vi "20.04.2025 class.vi"() -> ()   [LabVIEW 2020]
panel:
  in  "second subarray 3":dbl[][][](array[numeric])
  out "output array":dbl[](array[numeric])
  out "reversed array 2":dbl[](array[numeric])
  out "second subarray":dbl[](array[numeric])
  out "first subarray":dbl[](array[numeric])
  out "reversed array":dbl[](array[numeric])
  in  "Array":dbl[](array[numeric])
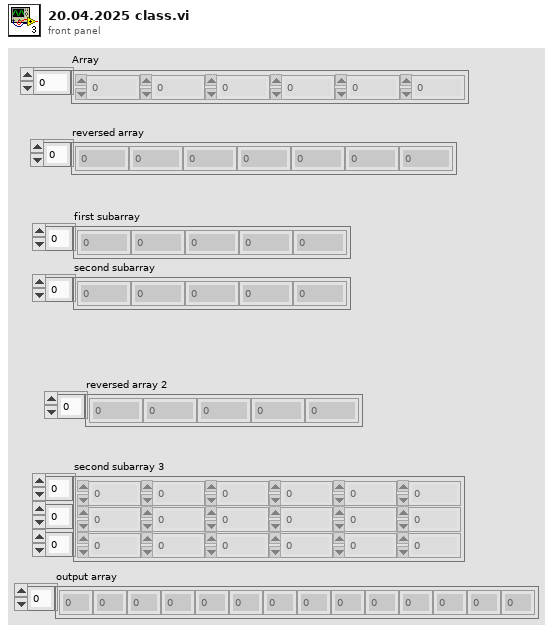
[diagram p1: front panel]
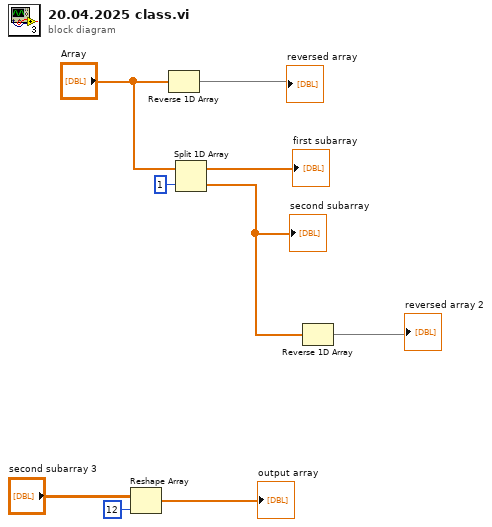
[diagram p0: block diagram]
diagram:
  n1 = Reshape Array "Reshape Array"("second subarray 3", 12 ("dimension size")) -> (→"output array":dbl[])
  n2 = Reverse 1D Array(array="Array") -> (reversed array=→"reversed array":dbl[])
  n3 = Split 1D Array(array="Array", index=1) -> (first subarray=→"first subarray":dbl[], second subarray=w4:dbl[])
  "second subarray" <- w4
  n4 = Reverse 1D Array(array=w4) -> (reversed array=→"reversed array 2":dbl[])
